vi "计算器20220522.vi"() -> ()   [LabVIEW 2010]
panel:
  out "临时操作存储":string
  out "临时输入存储":string
  out "显示":string
  out "结果":string
  out "输入2":string
  out "输入1":string
  in  "操作/":bool
  in  "操作*":bool
  in  "操作-":bool
  in  "操作+":bool
  in  "等于=":bool
  in  "清除":bool
  in  "小数点.":bool
  in  "数字0":bool
  in  "±号":bool
  in  "数字9":bool
  in  "数字8":bool
  in  "数字7":bool
  in  "数字6":bool
  in  "数字5":bool
  in  "数字4":bool
  in  "数字3":bool
  in  "数字2":bool
  in  "数字1":bool
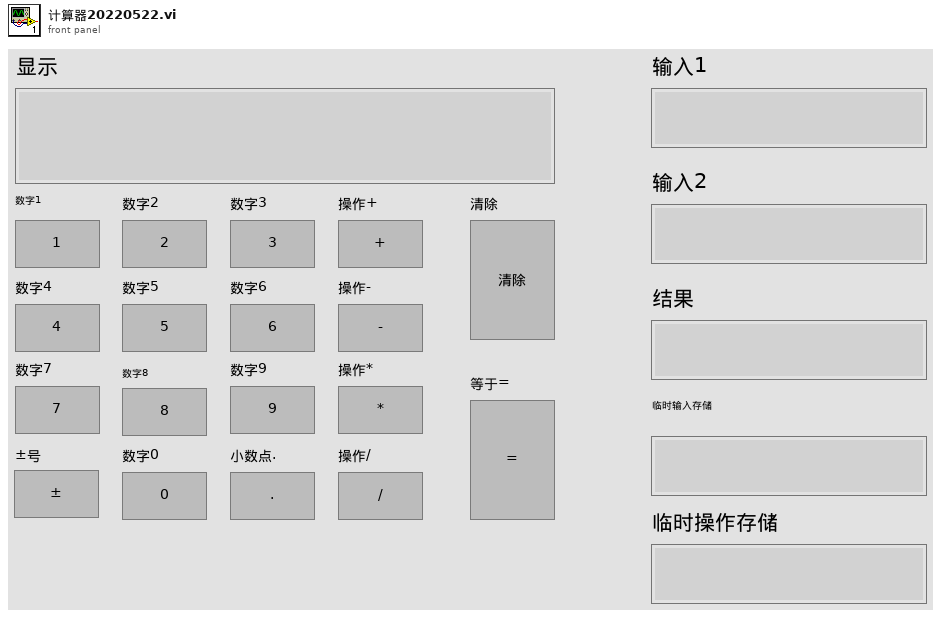
[diagram p1: front panel]
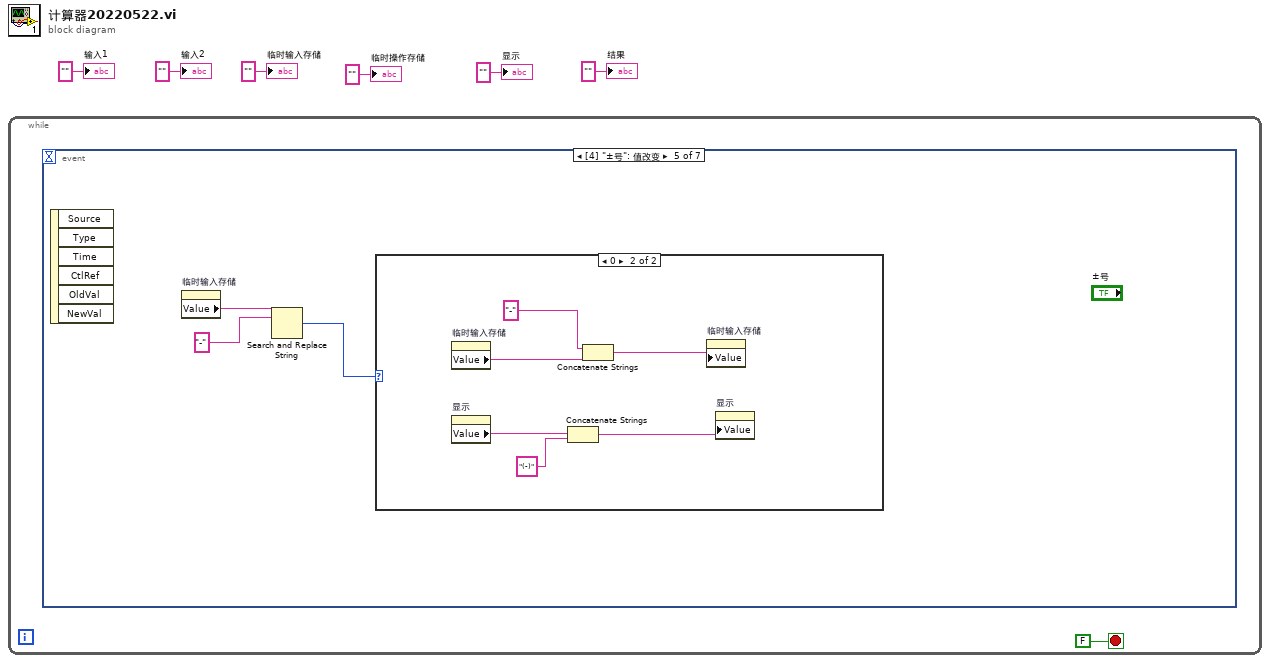
[diagram p0: block diagram]
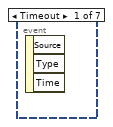
[diagram p2: hidden frame]
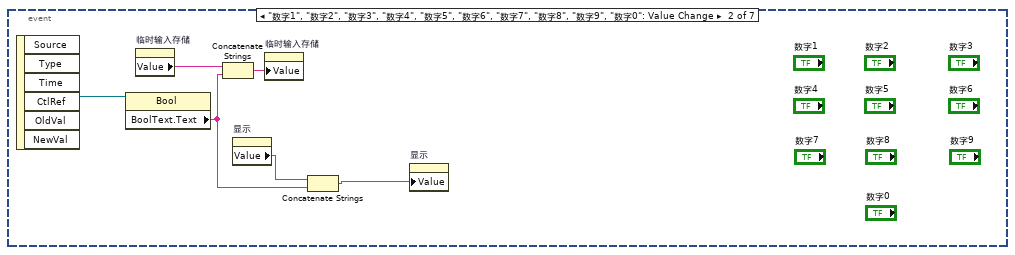
[diagram p3: hidden frame]
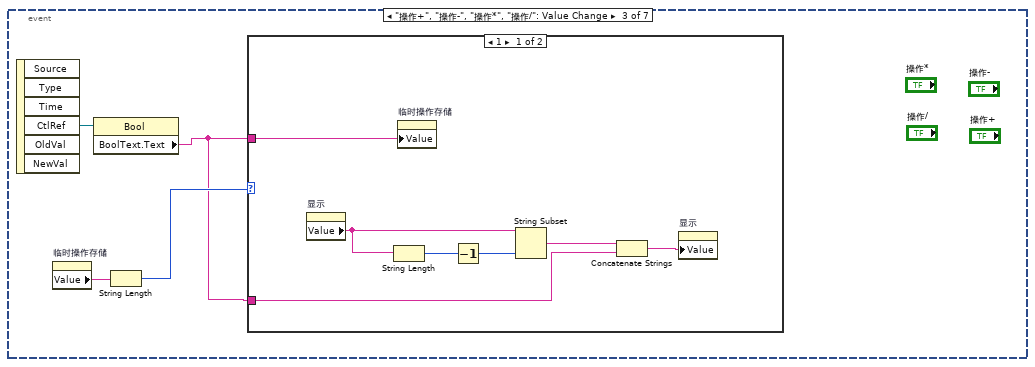
[diagram p4: hidden frame]
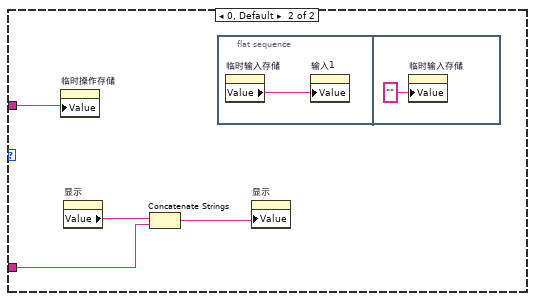
[diagram p5: hidden frame]
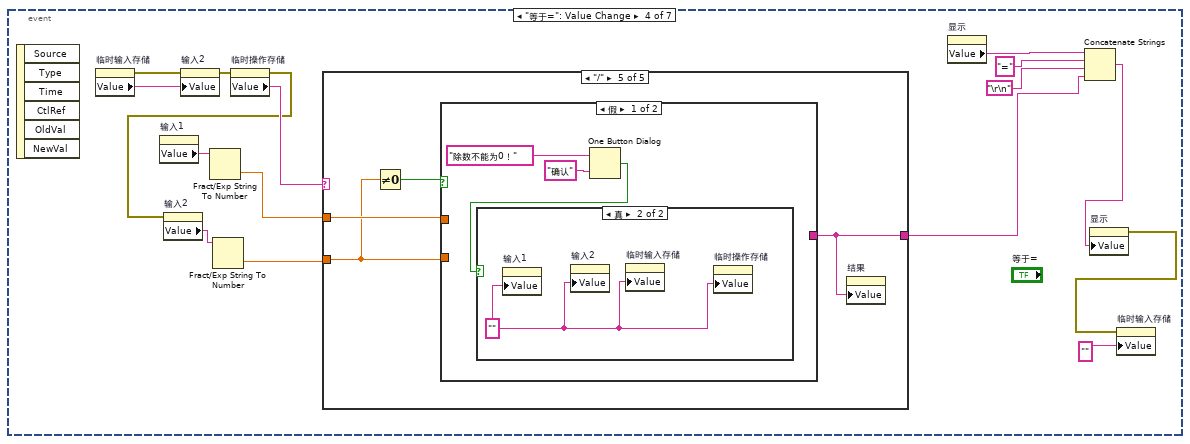
[diagram p6: hidden frame]
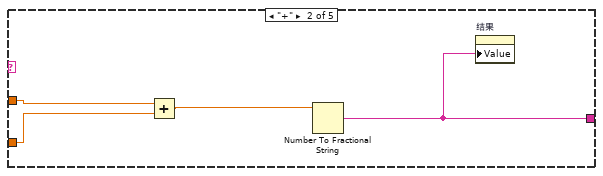
[diagram p8: hidden frame]
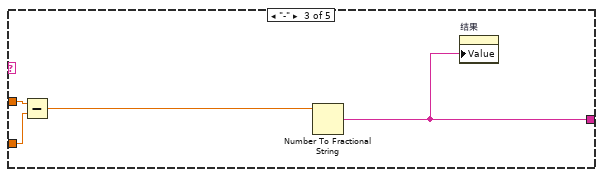
[diagram p9: hidden frame]
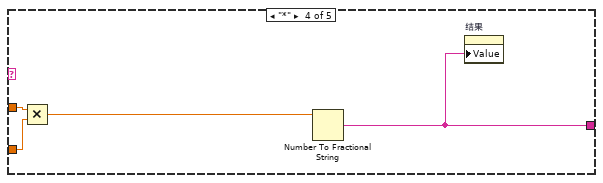
[diagram p10: hidden frame]
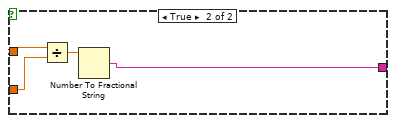
[diagram p12: hidden frame]
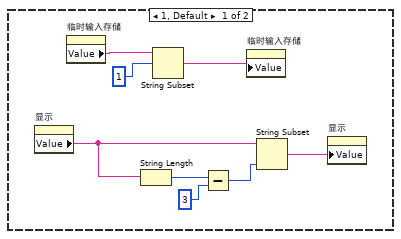
[diagram p13: hidden frame]
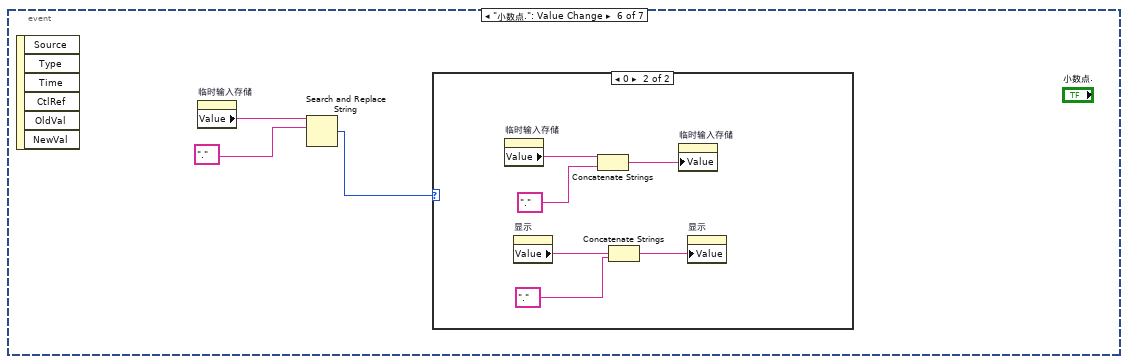
[diagram p14: hidden frame]
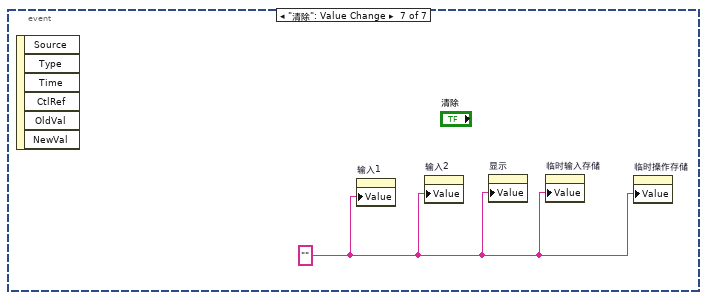
[diagram p16: hidden frame]
diagram:
  n1 = while {
    stop <- FALSE stop-if-true
    n2 = event shown="[4] \"±号\": 值改变" {
      selector: _ -> [_ _ _ _ _ _ _]
      dyn-events: _ -> [_ _ _ _ _ _ _]
      timeout: _ -> [_ _ _ _ _ _ _]
      event Timeout {
        n3 = event-data() -> ()  [unwired: 1 in, 3 out]
      }
      event "数字1", "数字2", "数字3", "数字4", "数字5", "数字6", "数字7", "数字8", "数字9", "数字0": Value Change {
        n4 = event-data() -> ("CtlRef"=w13:refnum<vi>)  [unwired: 1 in, 5 out]
        n5 = property class="Bool"(reference=w13) -> ("BoolText.Text"=w8:string)  [unwired: 1 in, 2 out]
        n6 = property on="临时输入存储" class="Str"() -> ("Value"=w12:string)  [unwired: 2 in, 2 out]
        n7 = Concatenate Strings(w12, w8) -> (w11:string)
        n8 = property on="显示" class="Str"() -> ("Value"=w10:string)  [unwired: 2 in, 2 out]
        n9 = property on="临时输入存储" class="Str"("Value"=w11) -> ()  [unwired: 2 in, 2 out]
        n10 = Concatenate Strings(w10, w8) -> (w9:string)
        n11 = property on="显示" class="Str"("Value"=w9) -> ()  [unwired: 2 in, 2 out]
      }
      event "操作+", "操作-", "操作*", "操作/": Value Change {
        n12 = event-data() -> ("CtlRef"=w17:refnum<vi>)  [unwired: 1 in, 5 out]
        n13 = property on="临时操作存储" class="Str"() -> ("Value"=w16:string)  [unwired: 2 in, 2 out]
        n14 = property class="Bool"(reference=w17) -> ("BoolText.Text"=w14:string)  [unwired: 1 in, 2 out]
        n15 = String Length(string=w16) -> (length=w15:i32)
        n16 = case shown="1" w15 {
          tunnel: w14 -> [w20 w27]
          tunnel: w14 -> [w18 w25]
          frame 1 {
            n17 = property on="显示" class="Str"() -> ("Value"=w22:string)  [unwired: 2 in, 2 out]
            n18 = String Length(string=w22) -> (length=w24:i32)
            n19 = property on="临时操作存储" class="Str"("Value"=w20) -> ()  [unwired: 2 in, 2 out]
            n20 = Decrement(x=w24) -> (x-1=w23:i32)
            n21 = String Subset(string=w22, length (rest)=w23) -> (substring=w21:string)  [unwired: 1 in]
            n22 = Concatenate Strings(w21, w18) -> (w19:string)
            n23 = property on="显示" class="Str"("Value"=w19) -> ()  [unwired: 2 in, 2 out]
          }
          frame 0, Default {
            n24 = property on="临时操作存储" class="Str"("Value"=w27) -> ()  [unwired: 2 in, 2 out]
            n25 = property on="显示" class="Str"() -> ("Value"=w26:string)  [unwired: 2 in, 2 out]
            n26 = Concatenate Strings(w26, w25) -> (w28:string)
            n27 = flat-sequence {
              frame #0 {
                n28 = property on="临时输入存储" class="Str"() -> ("Value"=w29:string)  [unwired: 2 in, 2 out]
                n29 = property on="输入1" class="Str"("Value"=w29) -> ()  [unwired: 2 in, 2 out]
              }
              frame #1 {
                n30 = property on="临时输入存储" class="Str"("Value"="" ("临时输入存储")) -> ()  [unwired: 2 in, 2 out]
              }
            }
            n31 = property on="显示" class="Str"("Value"=w28) -> ()  [unwired: 2 in, 2 out]
          }
        }
      }
      event "等于=": Value Change {
        n32 = event-data() -> ()  [unwired: 1 in, 6 out]
        n33 = property on="临时输入存储" class="Str"() -> (error out=w44:errorcluster, "Value"=w46:string)  [unwired: 2 in, 1 out]
        n34 = property on="输入1" class="Str"() -> ("Value"=w42:string)  [unwired: 2 in, 2 out]
        n35 = property on="输入2" class="Str"(error in=w44, "Value"=w46) -> (error out=w43:errorcluster)  [unwired: 1 in, 1 out]
        n36 = Fract/Exp String To Number(string=w42) -> (number=w39:dbl)  [unwired: 3 in, 1 out]
        n37 = property on="临时操作存储" class="Str"(error in=w43) -> (error out=w40:errorcluster, "Value"=w45:string)  [unwired: 1 in, 1 out]
        n38 = property on="输入2" class="Str"(error in=w40) -> ("Value"=w41:string)  [unwired: 1 in, 2 out]
        n39 = Fract/Exp String To Number(string=w41) -> (number=w38:dbl)  [unwired: 3 in, 1 out]
        n40 = case shown="\"/\"" w45 {
          tunnel: w39 -> [_ w49 w53 w57 w62]
          tunnel: w38 -> [_ w48 w52 w56 w61]
          tunnel: [_ w47 w51 w55 w59] -> w33
          frame "假", Default {
          }
          frame "+" {
            n41 = Add(x=w49, y=w48) -> (x+y=w50:dbl)
            n42 = Number To Fractional String(number=w50) -> (F-format string=w47:string)  [unwired: 3 in]
            n43 = property on="结果" class="Str"("Value"=w47) -> ()  [unwired: 2 in, 2 out]
          }
          frame "-" {
            n44 = Subtract(x=w53, y=w52) -> (x-y=w54:dbl)
            n45 = Number To Fractional String(number=w54) -> (F-format string=w51:string)  [unwired: 3 in]
            n46 = property on="结果" class="Str"("Value"=w51) -> ()  [unwired: 2 in, 2 out]
          }
          frame "*" {
            n47 = Multiply(x=w57, y=w56) -> (x*y=w58:dbl)
            n48 = Number To Fractional String(number=w58) -> (F-format string=w55:string)  [unwired: 3 in]
            n49 = property on="结果" class="Str"("Value"=w55) -> ()  [unwired: 2 in, 2 out]
          }
          frame "/" {
            n50 = Not Equal To 0?(x=w61) -> (x != 0?=w60:bool)
            n51 = case shown="假" w60 {
              tunnel: w62 -> [_ w70]
              tunnel: w61 -> [_ w69]
              tunnel: [_ w67] -> w59
              frame False {
                n52 = One Button Dialog(message="除数不能为0！" ("消息"), button name ("OK")="确认" ("消息")) -> (true=w63:bool)
                n53 = case shown="真" w63 {
                  frame False {
                  }
                  frame True {
                    w66 = "" ("临时输入存储")
                    n54 = property on="输入1" class="Str"("Value"=w66) -> ()  [unwired: 2 in, 2 out]
                    n55 = property on="输入2" class="Str"("Value"=w66) -> ()  [unwired: 2 in, 2 out]
                    n56 = property on="临时输入存储" class="Str"("Value"=w66) -> ()  [unwired: 2 in, 2 out]
                    n57 = property on="临时操作存储" class="Str"("Value"=w66) -> ()  [unwired: 2 in, 2 out]
                  }
                }
              }
              frame True {
                n58 = Divide(x=w70, y=w69) -> (x/y=w68:dbl)
                n59 = Number To Fractional String(number=w68) -> (F-format string=w67:string)  [unwired: 3 in]
              }
            }
            n60 = property on="结果" class="Str"("Value"=w59) -> ()  [unwired: 2 in, 2 out]
          }
        }
        n61 = property on="显示" class="Str"() -> ("Value"=w37:string)  [unwired: 2 in, 2 out]
        n62 = Concatenate Strings(w37, "=" ("输入2"), "\r\n", w33) -> (w34:string)
        n63 = property on="显示" class="Str"("Value"=w34) -> (error out=w32:errorcluster)  [unwired: 2 in, 1 out]
        n64 = property on="临时输入存储" class="Str"(error in=w32, "Value"="" ("临时输入存储")) -> ()  [unwired: 1 in, 2 out]
      }
      event "±号": Value Change {
        n65 = event-data() -> ()  [unwired: 1 in, 6 out]
        n66 = property on="临时输入存储" class="Str"() -> ("Value"=w73:string)  [unwired: 2 in, 2 out]
        n67 = Search and Replace String(input string=w73, search string="-" ("搜索字符串")) -> (number of replacements=w71:i32)  [unwired: 6 in, 3 out]
        n68 = case shown="0" w71 {
          frame 1, Default {
            n69 = property on="显示" class="Str"() -> ("Value"=w77:string)  [unwired: 2 in, 2 out]
            n70 = property on="临时输入存储" class="Str"() -> ("Value"=w81:string)  [unwired: 2 in, 2 out]
            n71 = String Length(string=w77) -> (length=w79:i32)
            n72 = String Subset(string=w81, offset (0)=1 ("偏移量(0)")) -> (substring=w80:string)  [unwired: 1 in]
            n73 = Subtract(x=w79, y=3 ("x-y")) -> (x-y=w75:i32)
            n74 = property on="临时输入存储" class="Str"("Value"=w80) -> ()  [unwired: 2 in, 2 out]
            n75 = String Subset(string=w77, length (rest)=w75) -> (substring=w76:string)  [unwired: 1 in]
            n76 = property on="显示" class="Str"("Value"=w76) -> ()  [unwired: 2 in, 2 out]
          }
          frame 0 {
            n77 = property on="临时输入存储" class="Str"() -> ("Value"=w86:string)  [unwired: 2 in, 2 out]
            n78 = property on="显示" class="Str"() -> ("Value"=w82:string)  [unwired: 2 in, 2 out]
            n79 = Concatenate Strings(w82, "(-)" ("字符串")) -> (w84:string)
            n80 = Concatenate Strings("-" ("字符串"), w86) -> (w85:string)
            n81 = property on="临时输入存储" class="Str"("Value"=w85) -> ()  [unwired: 2 in, 2 out]
            n82 = property on="显示" class="Str"("Value"=w84) -> ()  [unwired: 2 in, 2 out]
          }
        }
      }
      event "小数点.": Value Change {
        n83 = event-data() -> ()  [unwired: 1 in, 6 out]
        n84 = property on="临时输入存储" class="Str"() -> ("Value"=w89:string)  [unwired: 2 in, 2 out]
        n85 = Search and Replace String(input string=w89, search string="." ("搜索字符串")) -> (number of replacements=w88:i32)  [unwired: 6 in, 3 out]
        n86 = case shown="0" w88 {
          frame 1, Default {
          }
          frame 0 {
            n87 = property on="临时输入存储" class="Str"() -> ("Value"=w96:string)  [unwired: 2 in, 2 out]
            n88 = property on="显示" class="Str"() -> ("Value"=w93:string)  [unwired: 2 in, 2 out]
            n89 = Concatenate Strings(w96, "." ("搜索字符串")) -> (w94:string)
            n90 = Concatenate Strings(w93, "." ("搜索字符串")) -> (w91:string)
            n91 = property on="临时输入存储" class="Str"("Value"=w94) -> ()  [unwired: 2 in, 2 out]
            n92 = property on="显示" class="Str"("Value"=w91) -> ()  [unwired: 2 in, 2 out]
          }
        }
      }
      event "清除": Value Change {
        w97 = "" ("临时输入存储")
        n93 = event-data() -> ()  [unwired: 1 in, 6 out]
        n94 = property on="输入1" class="Str"("Value"=w97) -> ()  [unwired: 2 in, 2 out]
        n95 = property on="输入2" class="Str"("Value"=w97) -> ()  [unwired: 2 in, 2 out]
        n96 = property on="显示" class="Str"("Value"=w97) -> ()  [unwired: 2 in, 2 out]
        n97 = property on="临时输入存储" class="Str"("Value"=w97) -> ()  [unwired: 2 in, 2 out]
        n98 = property on="临时操作存储" class="Str"("Value"=w97) -> ()  [unwired: 2 in, 2 out]
      }
    }
  }
  "输入1" <- "" ("输入2")
  "输入2" <- "" ("输入2")
  "显示" <- "" ("输入2")
  "结果" <- "" ("输入2")
  "临时输入存储" <- "" ("输入2")
  "临时操作存储" <- "" ("输入2")
